vi "disable_all.vi"(8 "error in (no error)":errorcluster caption="错误输入（无错误）", 11 "MotorSystem 输入":refnum<class "MotorSystem.lvclass">) -> (0 "error out":errorcluster caption="错误输出", 3 "MotorSystem 输出":refnum<class "MotorSystem.lvclass">)   [LabVIEW 2016, in "MotionControl_UFO_3DOF.lvlib" / "MotorSystem.lvclass"]
uses:
  <userlib>/MotionControl_UFO_3DOF/MotorSystem/MotorSystem.lvclass
  <userlib>/MotionControl_UFO_3DOF/MotorSystem/MotorSystem.lvclass/MotorSystem.ctl
  <userlib>/MotionControl_UFO_3DOF/OneMotion/OneMotion.lvclass/OneMotion.ctl
  <userlib>/MotionControl_UFO_3DOF/OneMotion/OneMotion.lvclass
  <userlib>/UISimCanFunc_wrapper/UISimCanFunc_wrapper.lvlib
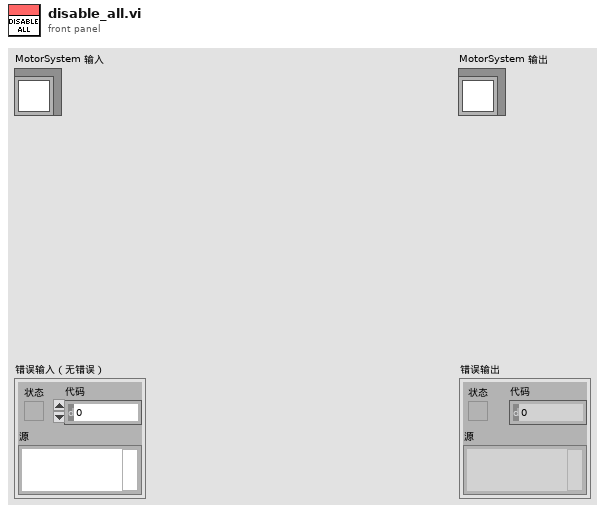
[diagram p1: front panel]
types:
  T1 = typedef "MotionControl_UFO_3DOF.lvlib/MotorSystem.lvclass/MotionCluster.ctl" = cluster{"OneMotion.lvclass":refnum<class "OneMotion.lvclass">, "connected?":bool, "default enabled?":bool, "enabled?":bool}
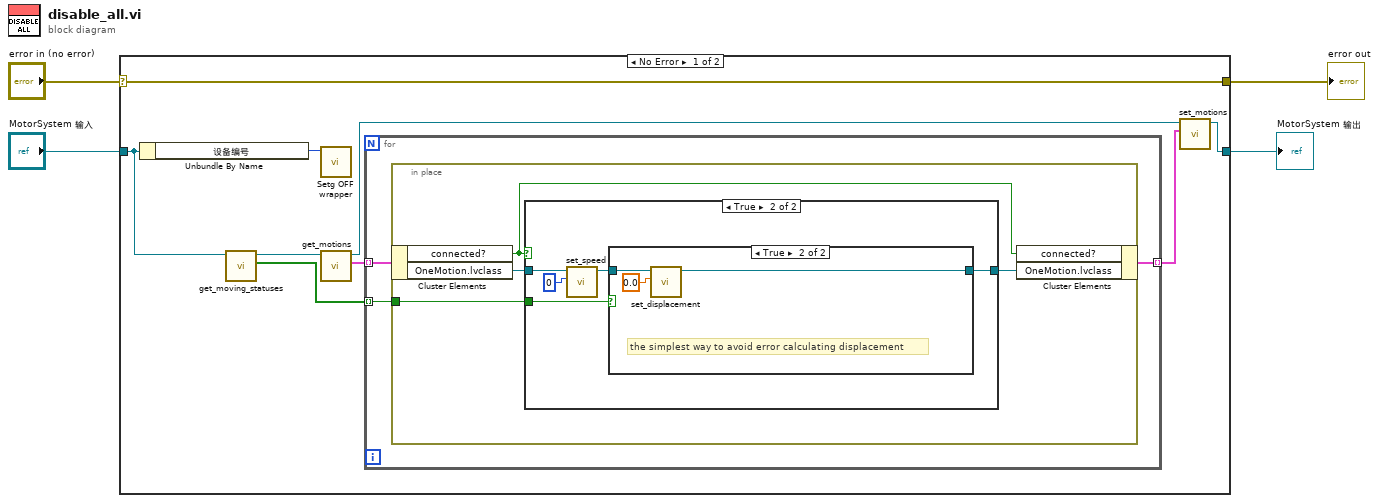
[diagram p0: block diagram]
diagram:
  n1 = case shown="No Error" "error in (no error)" {
    selector: "error in (no error)" -> [w13 w32]
    tunnel: [w13 w32] -> w3
    tunnel: [w8 w31] -> w1
    tunnel: "MotorSystem 输入" -> [w7 w31]
    frame No Error {
      n2 = Unbundle By Name(w7) -> ("设备编号"=w12:u32)
      n3 = call <userlib>:"get_moving_statuses.vi"("MotorSystem输入"=w7) -> ("moving?"=w5:bool[], "MotorSystem输出"=w6:refnum<class "MotorSystem.lvclass">)  [unwired: 8 in, 1 out]
      n4 = call <userlib>:"Setg OFF wrapper.vi"("dwDevIndex"=w12) -> ()  [unwired: 9 in, 2 out]
      n5 = call <userlib>:"get_motions.vi"("MotorSystem输入"=w6) -> ("motions"=w11:T1[], "MotorSystem输出"=w10:refnum<class "MotorSystem.lvclass">)  [unwired: 8 in, 1 out]
      n6 = for {
        tunnel: w11 -> [w16] mode=indexing
        tunnel: [w15] -> w9 mode=indexing
        tunnel: w5 -> [w14] mode=indexing
        n7 = in-place {
          in-place-border: w14 -> [w20]
          n8 = in-place-cluster #1(w16) -> ("connected?"=w17:bool, "OneMotion.lvclass"=w19:refnum<class "OneMotion.lvclass">)
          n9 = case shown="True" w17 {
            tunnel: w20 -> [_ w26]
            tunnel: w19 -> [w21 w25]
            tunnel: [w21 w22] -> w18
            frame False {
            }
            frame True {
              n10 = call-dynamic "set_speed.vi"("speed"=0, "OneMotion 输入"=w25) -> ("OneMotion 输出"=w23:refnum<class "OneMotion.lvclass">)  [unwired: 8 in, 1 out]
              n11 = case shown="True" w26 {
                tunnel: w23 -> [w27 w30]
                tunnel: [w27 w29] -> w22
                frame False {
                }
                frame True {
                  # "the simplest way to avoid error calculating displacement"
                  n12 = call <userlib>:"set_displacement.vi"("displacement"=0.0, "OneMotion输入"=w30) -> ("OneMotion输出"=w29:refnum<class "OneMotion.lvclass">)  [unwired: 8 in, 1 out]
                }
              }
            }
          }
          n13 = in-place-cluster #1("connected?"=w17, "OneMotion.lvclass"=w18) -> (w15:T1)
        }
      }
      n14 = call <userlib>:"set_motions.vi"("motions"=w9, "MotorSystem输入"=w10) -> ("MotorSystem输出"=w8:refnum<class "MotorSystem.lvclass">)  [unwired: 8 in, 1 out]
    }
    frame Error {
    }
  }
  "error out" <- w3
  "MotorSystem 输出" <- w1
